vi "New Extended Command.vi"(0 "RFFE Extended Command in":refnum<class "RFFE Extended Command.lvclass">, 1 "Alias":string, 5 "Slave Address":T3=12 format="%02x", 7 "Register Address":T2 format="%02x", 9 "Register Data":T1[](array[typedef]) format="%02x", 11 "error in (no error)":errorcluster) -> (4 "RFFE Extended Command out":refnum<class "RFFE Extended Command.lvclass">, 15 "error out":errorcluster)   [LabVIEW 2018, in "MIPI RFFE API.lvlib" / "RFFE Extended Command.lvclass"]
uses:
  RFFE Extended Command.lvclass
  C:/Users/semoore/Projects/mipi-rffe-labview-oop/Command/RFFE Command.lvclass
  Slave Address.ctl
  Register Address.ctl
  Register Data.ctl
  RFFE Extended Command.lvclass/RFFE Extended Command.ctl
  Set Register Data.vi
  Command/RFFE Command.lvclass
  MIPI RFFE API.lvlib
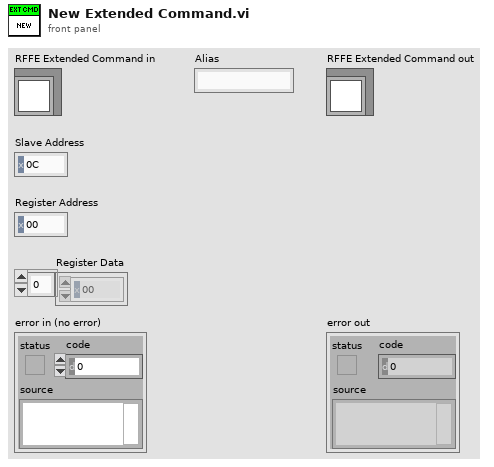
[diagram p1: front panel]
types:
  T1 = typedef "MIPI RFFE API.lvlib/Register Data.ctl" = u8
  T2 = typedef "MIPI RFFE API.lvlib/Register Address.ctl" = u16
  T3 = typedef "MIPI RFFE API.lvlib/Slave Address.ctl" = u8
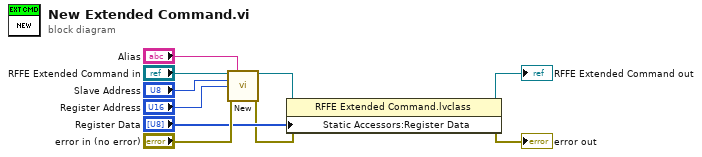
[diagram p0: block diagram]
diagram:
  n1 = call "New.vi"("RFFE Command in"="RFFE Extended Command in", "Alias"="Alias", "Slave Address"="Slave Address", "Register Address"="Register Address", "error in (no error)"="error in (no error)") -> ("RFFE Command out"=w3:refnum<class "RFFE Extended Command.lvclass">, "error out"=w2:errorcluster)  [unwired: 9 in]
  n2 = property class="RFFE Extended Command.lvclass"(reference=w3, error in=w2, "Static Accessors:Register Data"="Register Data") -> (reference out=→"RFFE Extended Command out":refnum<class "RFFE Extended Command.lvclass">, error out=→"error out":errorcluster)
